vi "QueueAndorCamOutToMainAndRoi.vi"(0 "Queue Andor0":refnum<queue>, 1 "Queue Andor1":refnum<queue>, 5 "error in (no error)":errorcluster) -> (14 "IntensityGraphAndor0":i32[][](graph), 15 "IntensityGraphAndor1":i32[][](graph), 19 "error out":errorcluster)   [LabVIEW 2011]
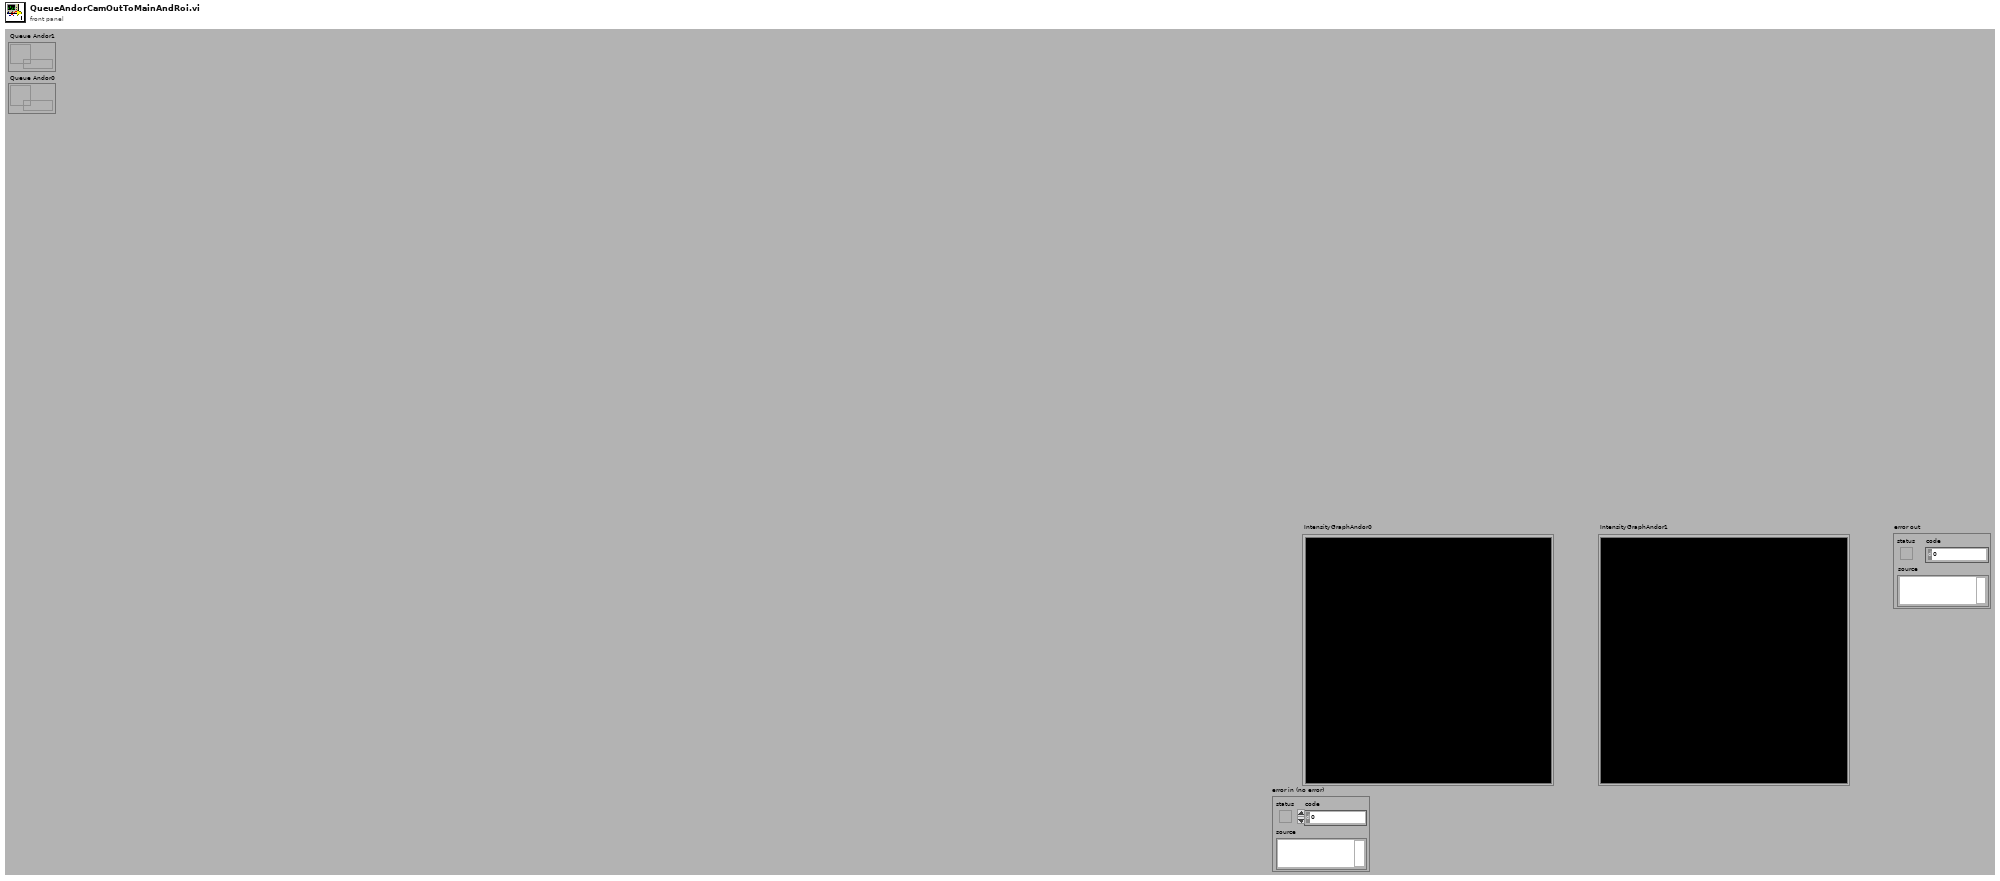
[diagram p1: front panel]
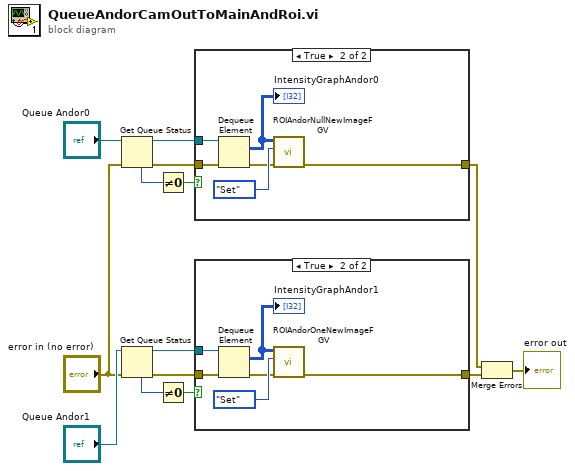
[diagram p0: block diagram]
diagram:
  n1 = Get Queue Status(queue="Queue Andor0", error in (no error)="error in (no error)") -> (queue out=w7:refnum<queue>, error out=w9:errorcluster, # elements in queue=w10:i32)  [unwired: 1 in, 5 out]
  n2 = Get Queue Status(queue="Queue Andor1", error in (no error)="error in (no error)") -> (queue out=w13:refnum<queue>, error out=w12:errorcluster, # elements in queue=w14:i32)  [unwired: 1 in, 5 out]
  n3 = Not Equal To 0?(x=w10) -> (x != 0?=w8:bool)
  n4 = Not Equal To 0?(x=w14) -> (x != 0?=w11:bool)
  n5 = case shown="True" w8 {
    tunnel: w9 -> [w15 w21]
    tunnel: [w15 w17] -> w3
    tunnel: w7 -> [_ w20]
    frame False {
    }
    frame True {
      n6 = Dequeue Element(queue=w20, error in (no error)=w21) -> (element=w16:i32[][], error out=w18:errorcluster)  [unwired: 1 in, 2 out]
      "IntensityGraphAndor0" <- w16
      n7 = call "ROIAndorNullNewImageFGV.vi"("error in"=w18, "FGV_Control"=enum16{"Set", "Get"}."Set", "IntensityGraphAndor0 in"=w16) -> ("error out"=w17:errorcluster)  [unwired: 7 in, 1 out]
    }
  }
  n8 = case shown="True" w11 {
    tunnel: w12 -> [w22 w28]
    tunnel: [w22 w25] -> w2
    tunnel: w13 -> [_ w27]
    frame False {
    }
    frame True {
      n9 = Dequeue Element(queue=w27, error in (no error)=w28) -> (element=w23:i32[][], error out=w24:errorcluster)  [unwired: 1 in, 2 out]
      "IntensityGraphAndor1" <- w23
      n10 = call "ROIAndorOneNewImageFGV.vi"("error in"=w24, "FGV_Control"=enum16{"Set", "Get"}."Set", "IntensityGraphAndor1 set"=w23) -> ("error out"=w25:errorcluster)  [unwired: 7 in, 1 out]
    }
  }
  n11 = Merge Errors(w3, w2) -> (→"error out":errorcluster)
